vi "Ch1-Ex2.vi"() -> ()   [LabVIEW 2018]
panel:
  in  "K":dbl
  out "J":dbl
  in  "I":dbl
  # "Implementation 1"
  # "Implementation 2"
  # "Implementation 3"
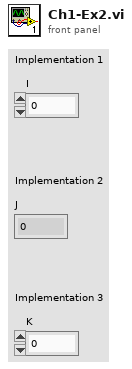
[diagram p1: front panel]
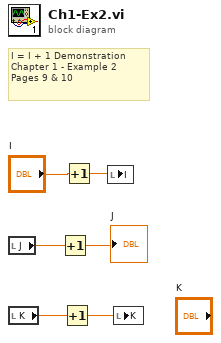
[diagram p0: block diagram]
diagram:
  # "I = I + 1 Demonstration\nChapter 1 - Example 2\nPages 9 & 10"
  n1 = local read "J"() -> (w4:dbl)
  n2 = local read "K"() -> (w2:dbl)
  n3 = Increment(x=w4) -> (x+1=→"J":dbl)
  n4 = Increment(x=w2) -> (x+1=w1:dbl)
  n5 = Increment(x="I") -> (x+1=w5:dbl)
  n6 = local write "I"(w5) -> ()
  n7 = local write "K"(w1) -> ()
